vi "Deploy_DisplayImageInfo.vi"(8 "error in (no error)":errorcluster, 11 "AppImage Properties":T1) -> (0 "error out":errorcluster, 2 "Cancelled?":bool)   [LabVIEW 2021]
uses:
  TypeDefs/AppImageProperties.ctl
  TypeDefs/FPGA_Properties_Element.ctl
panel:
  out "Blacklist":string[](array[string])=["/var/lib/zerotier-one/identity.public", "/var/lib/zerotier-one/identity.secret"] caption="File and Directory\nBlacklist"
  out "Version.Revision":u8
  out "Version.Minor":u8
  in  "Cancel":bool
  in  "RetireveImg":bool
  out "Version.Major":u8 caption="Version"
  out "Description":string
  out "Title":string
  # "Image Properties"
  # "."
  # "."
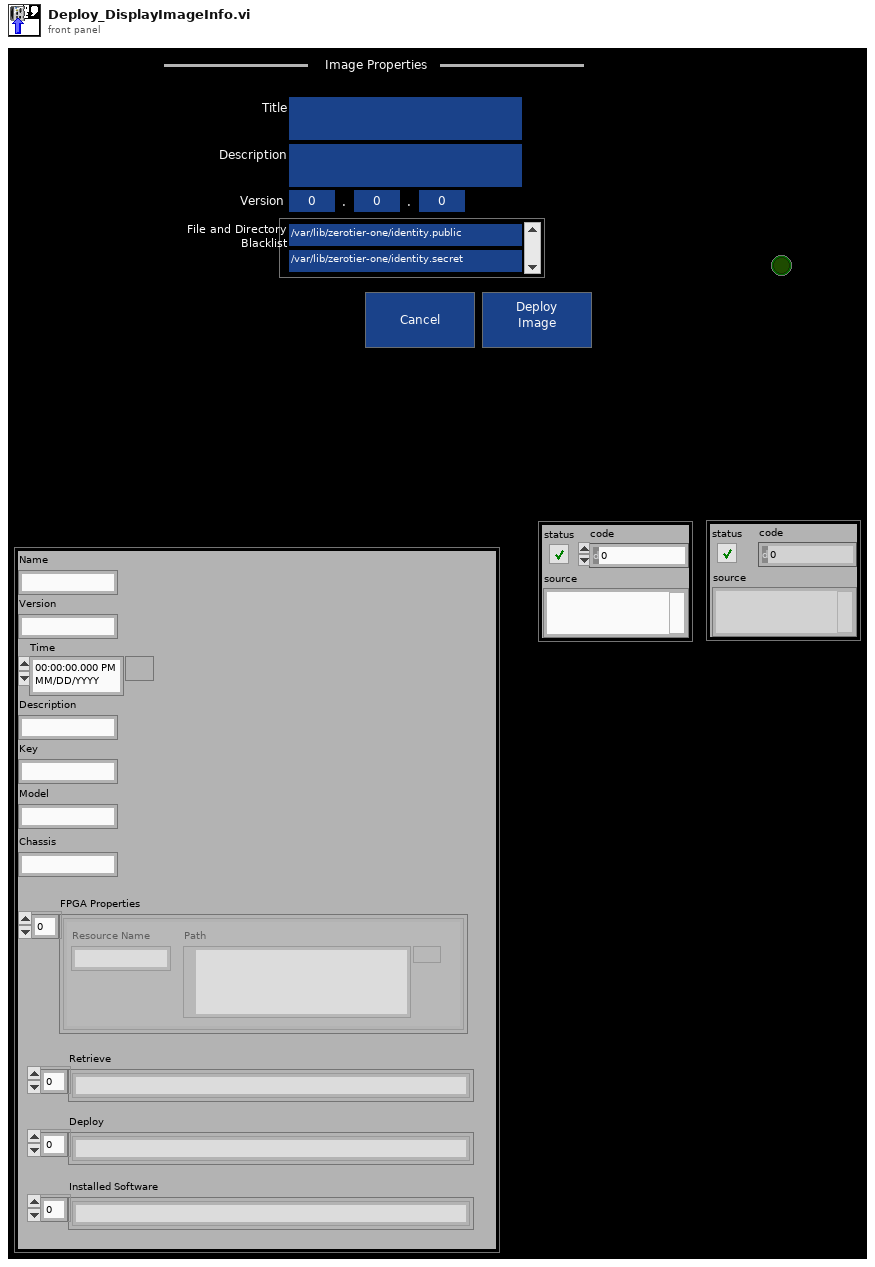
[diagram p1: front panel]
types:
  T1 = typedef "AppImageProperties.ctl" = cluster{"Name":string, "Version":string, "Time":timestamp, "Description":string, "Key":string, "Chassis":string, "FPGA Properties":T2[], "Model":string, "Retrieve":string[], "Deploy":string[], "Installed Software":string[]}
  T2 = typedef "FPGA_Properties_Element.ctl" = cluster{"Resource Name":string, "Path":path}
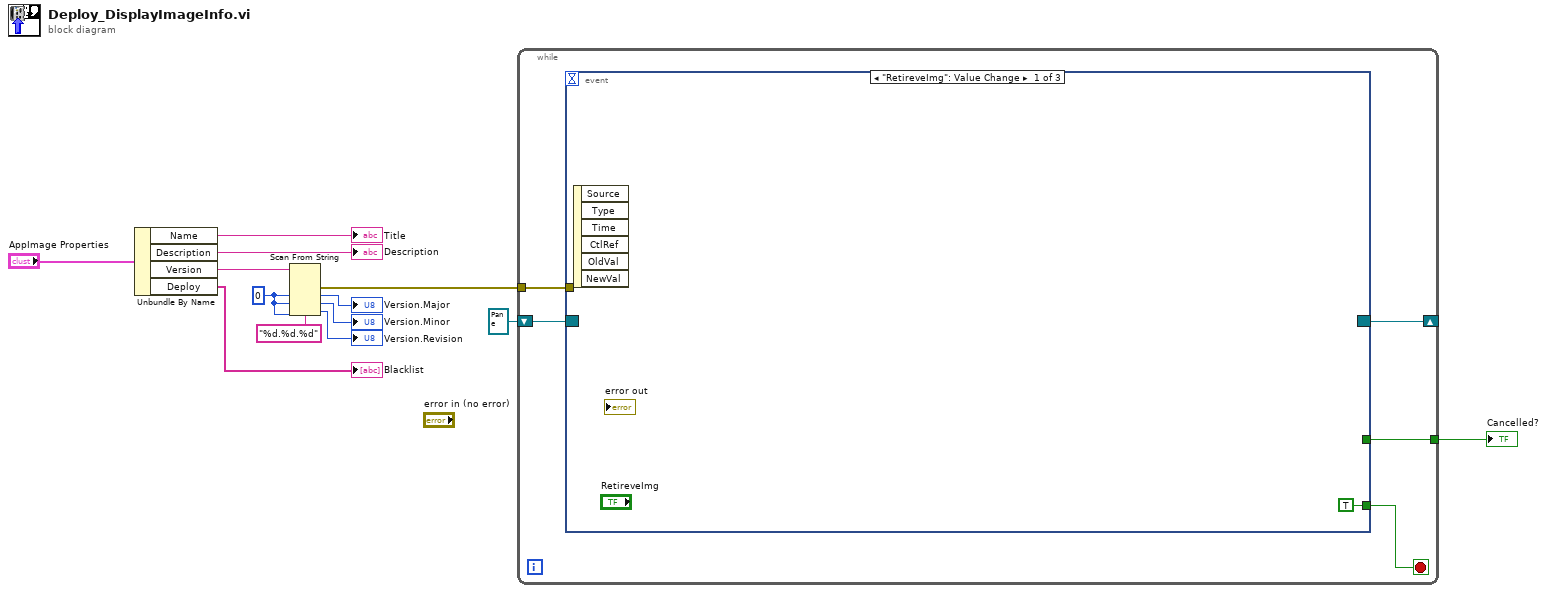
[diagram p0: block diagram]
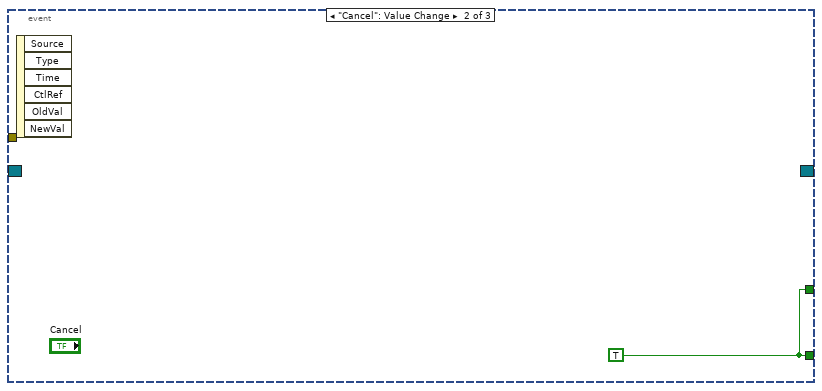
[diagram p2: hidden frame]
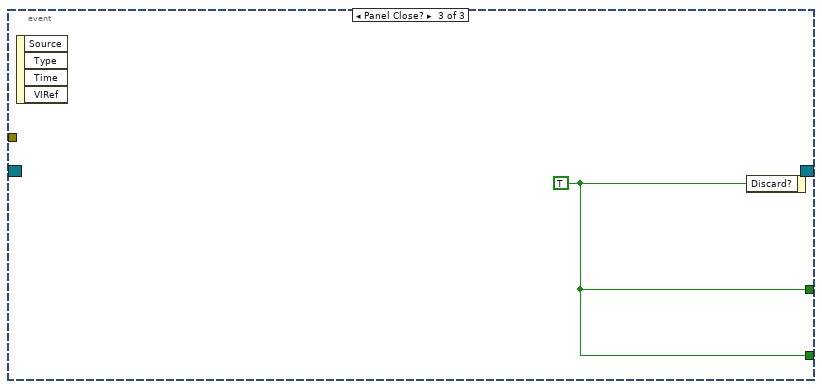
[diagram p3: hidden frame]
diagram:
  w10 = u8 0 ("default value 1")
  n1 = Unbundle By Name("AppImage Properties") -> ("Name"=→"Title":string, "Description"=→"Description":string, "Version"=w11:string, "Deploy"=→"Blacklist":string[])
  n2 = Scan From String(format string="%d.%d.%d", input string=w11, default 1=w10, default 2=w10, default 3=w10) -> (error out=w9:errorcluster, output 1=→"Version.Major":u8, output 2=→"Version.Minor":u8, output 3=→"Version.Revision":u8)  [unwired: 2 in, 2 out]
  n3 = while {
    tunnel: w9 -> [w18]
    shift-right: [w16] -> _
    shift-left: refnum<event-registration> refnum ("Event Registration Refnum") -> [w15]
    tunnel: [w14] -> w7
    stop <- w17 stop-if-true
    n4 = event shown="[0] \"RetireveImg\": Value Change" {
      selector: w15 -> [_ _ _]
      dyn-events: [_ _ _] -> w16
      timeout: _ -> [_ _ _]
      tunnel: w18 -> [_ _ _]
      tunnel: [TRUE ("Discard?") w20 w21] -> w17
      tunnel: [_ w20 w21] -> w14
      event "RetireveImg": Value Change {
        n5 = event-data() -> ()  [unwired: 1 in, 6 out]
      }
      event "Cancel": Value Change {
        w20 = TRUE
        n6 = event-data() -> ()  [unwired: 1 in, 6 out]
      }
      event Panel Close? {
        w21 = TRUE ("Discard?")
        n7 = event-data() -> ()  [unwired: 1 in, 4 out]
        n8 = event-data("Discard?"=w21) -> ()  [unwired: 1 in, 1 out]
      }
    }
  }
  "Cancelled?" <- w7
